vi "BreakfastMenuIterator_Create.vi"(8 "Error In":errorcluster, 10 "Items":variant[](array[variant]), 11 "reference in":refnum<class "BreakfastMenuIterator.lvclass">) -> (0 "Error Out":errorcluster, 3 "reference out":refnum<class "BreakfastMenuIterator.lvclass">)   [LabVIEW 2020, in "BreakfastMenuIterator.lvclass"]
uses:
  BreakfastMenuIterator.lvclass
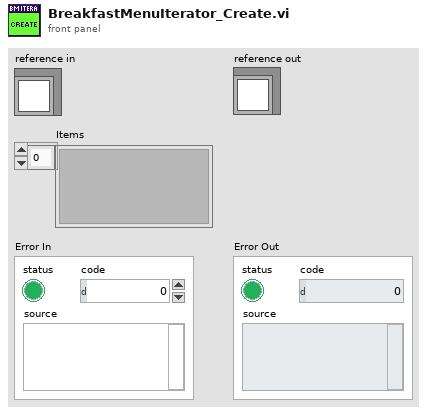
[diagram p1: front panel]
types:
  T1 = typedef "BreakfastMenuIterator.lvclass/ObjectAttributes.ctl" = cluster{"_count":i32, "_items":variant[]}
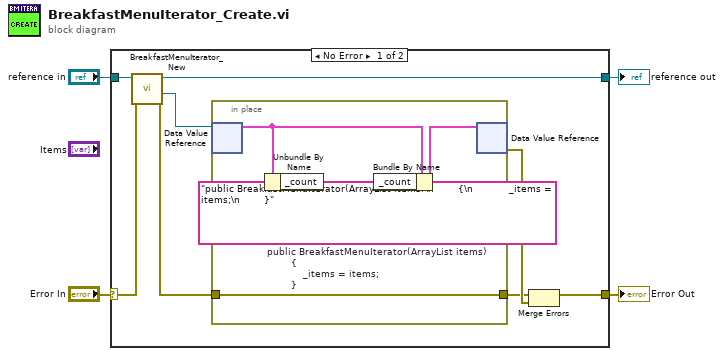
[diagram p0: block diagram]
diagram:
  (unwired) "public BreakfastMenuIterator(ArrayList items)\n        {\n            _items = items;\n        }"  # public BreakfastMenuIterator(ArrayList items)         {             _items = items;         }
  n1 = case shown="No Error" "Error In" {
    selector: "Error In" -> [w11 w18]
    tunnel: [w5 w18] -> w3
    tunnel: "reference in" -> [w12 w17]
    tunnel: [w10 w17] -> w1
    frame No Error {
      n2 = call "BreakfastMenuIterator_New.vi"("error in (no error)"=w11, "reference in"=w12) -> ("error out"=w7:errorcluster, "DVRRefOut"=w8:refnum<data-value>, "reference out"=w10:refnum<class "BreakfastMenuIterator.lvclass">)  [unwired: 6 in, 1 out]
      n3 = in-place {
        in-place-border: w7 -> [w13]
        in-place-border: [w13] -> w6
        n4 = in-place-dvr #1(w8) -> (w15:T1)  [unwired: 1 out]
        n5 = Unbundle By Name(w15) -> ("_count"=w14:i32)
        n6 = Bundle By Name(cluster=w15, "_count"=w14) -> (w16:T1)
        n7 = in-place-dvr #1(w16) -> (w9:errorcluster)  [unwired: 1 out]
      }
      n8 = Merge Errors(w6, w9) -> (w5:errorcluster)
    }
    frame Error {
      # "VI-TechBaseTemplate_Simple_4x4x4"
    }
  }
  "Error Out" <- w3
  "reference out" <- w1
